vi "ServiceClientExample.vi"() -> ()   [LabVIEW 2016]
uses:
  ROS/Code/Console/Servers/ServerSubs/TopicDef.ctl
  ROS/Code/SubVIs/_ROSDirection.ctl
  ROS/MessageBuilding/std_msgs/subs/i64Scalar.vi
  ROS/MessageParsing/std_msgs/subs/parse_u8_scalar.vi
  ROS/MessageParsing/std_msgs/subs/parse_i64_scalar.vi
panel:
  in  "stop":bool
  out "OK?":bool
  out "sum":i64
  in  "y":i64=2
  in  "x":i64=1
  in  "Service Call":bool
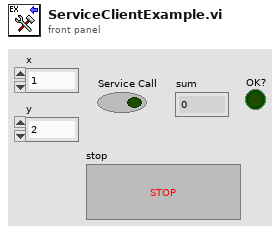
[diagram p1: front panel]
types:
  T1 = typedef "TopicDef.ctl" = cluster{"Topic":string, "Type":string, "Action":T2, "Update (ms)":u16, "queue size":u16}
  T2 = typedef "_ROSDirection.ctl" = enum16{"Node", "Publisher", "Subscriber", "ServiceClient", "ServiceProvider"}
  T3 = typedef "_ROSControl.ctl" = cluster{"topic port":u16, "Node":string, "topic":string, "type":string, "node port":u16, "error ":errorcluster, "Direction":T2, "Update (ms)":u16, "FIFO size":u16}
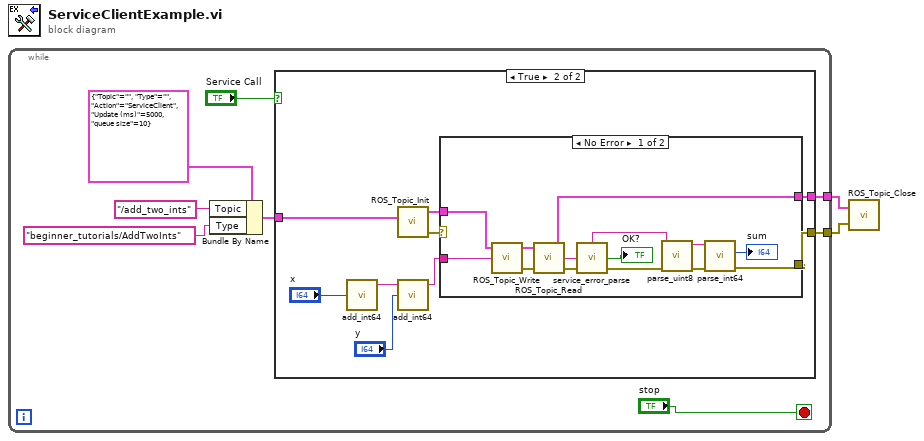
[diagram p0: block diagram]
diagram:
  n1 = while {
    tunnel: [w8] -> w2
    tunnel: [w7] -> w1
    stop <- "stop" stop-if-true
    n2 = Bundle By Name(cluster=T1 {"Topic"="", "Type"="", "Action"=enum."ServiceClient", "Update (ms)"=5000, "queue size"=10} ("Definitions"), "Topic"="/add_two_ints", "Type"="beginner_tutorials/AddTwoInts") -> (w3:T1)
    n3 = case shown="True" "Service Call" {
      tunnel: [_ w13] -> w8
      tunnel: [_ w12] -> w7
      tunnel: w3 -> [_ w11]
      frame False {
      }
      frame True {
        n4 = call-poly "add_int64.vi"("Numeric"="x") -> ("msg out"=w19:string)  [unwired: 4 in]
        n5 = call "ROS_Topic_Init.vi"("Definitions"=w11) -> ("ROS out"=w16:T3, "error out"=w15:errorcluster)  [unwired: 2 in]
        n6 = call-poly "add_int64.vi"("Numeric"="y", "msg in"=w19) -> ("msg out"=w14:string)  [unwired: 3 in]
        n7 = case shown="No Error" w15 {
          selector: w15 -> [_ w33]
          tunnel: w16 -> [w30 w34]
          tunnel: w14 -> [w29 _]
          tunnel: [w24 w34] -> w13
          tunnel: [w20 w33] -> w12
          frame No Error {
            n8 = call "ROS_Topic_Write.vi"("Msg in"=w29, "ROS in"=w30) -> ("error out"=w32:errorcluster, "ROS out"=w31:T3)  [unwired: 2 in]
            n9 = call "ROS_Topic_Read.vi"("error in (no error)"=w32, "ROS in"=w31) -> ("error out"=w28:errorcluster, "Reply"=w27:string, "ROS out"=w24:T3)  [unwired: 1 in]
            n10 = call "service_error_parse.vi"("error in (no error)"=w28, "Reply"=w27) -> ("error out"=w26:errorcluster, "OK?"=→"OK?":bool)  [unwired: 1 in, 1 out]
            n11 = call-poly "parse_uint8.vi"("error in"=w26, "msg in"=w27) -> ("error out"=w21:errorcluster, "msg out"=w23:string)  [unwired: 3 in, 1 out]
            n12 = call-poly "parse_int64.vi"("error in"=w21, "msg in"=w23) -> ("error out"=w20:errorcluster, "number"=→"sum":i64)  [unwired: 3 in, 1 out]
          }
          frame Error {
          }
        }
      }
    }
  }
  n13 = call "ROS_Topic_Close.vi"("error in"=w1, "ROS in"=w2) -> ()  [unwired: 2 in, 1 out]
